vi "Invert u16.vi"(11 "In (u16)":u16) -> (3 "Out (u16)":u16)   [LabVIEW 2015]
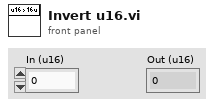
[diagram p1: front panel]
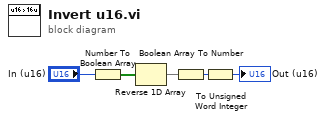
[diagram p0: block diagram]
diagram:
  n1 = Number To Boolean Array(number="In (u16)") -> (Boolean array=w5:bool[])
  n2 = Reverse 1D Array(array=w5) -> (reversed array=w4:bool[])
  n3 = Boolean Array To Number(Boolean array=w4) -> (number=w3:u32)
  n4 = To Unsigned Word Integer(number=w3) -> (unsigned 16bit integer=→"Out (u16)":u16)
